vi "Drive output parameters.vi"   [LabVIEW 2016]
uses:
  Robot Global Data.vi
types:
  T1 = enum16{"FL Drive Wheel", "FR Drive Wheel", "RL Drive Wheel", "RR Drive Wheel", "FL Steer Wheel", "FR Steer Wheel", "RL Steer Wheel", "RR Steer Wheel"}
  T2 = typedef "WPI_MotorControlDeviceRef.ctl" = cluster{"DeviceStatus":errorcluster, "Type":T3, "PWM":cluster{"PWM Channel":T4, "DeadBand":T5}, "CAN":cluster{"Device Number":u8, "SetOutput VI Ref":variant, "GetOutput VI Ref":variant, "Enable VI Ref":variant, "Disable VI Ref":variant, "Data":variant}, "Invert":bool}
  T3 = typedef "WPI_MotorControlType.ctl" = enum16{"PWM", "CAN"}
  T4 = typedef "FPGA_DIOPWMChannel.ctl" = enum8{"PWM 0", "PWM 1", "PWM 2", "PWM 3", "PWM 4", "PWM 5", "PWM 6", "PWM 7", "PWM 8", "PWM 9", "PWM MXP 0", "PWM MXP 1", "PWM MXP 2", "PWM MXP 3", "PWM MXP 4", "PWM MXP 5", "PWM MXP 6", "PWM MXP 7", "PWM MXP 8", "PWM MXP 9", "Invalid"}
  T5 = typedef "WPI_PWMDeadband.ctl" = cluster{"Name":string, "maxPositivePwm":i32, "minPositivePwm":i32, "centerPwm":i32, "maxNegativePwm":i32, "minNegativePwm":i32, "angularRange":u16}
  T6 = typedef "WPI_CANTalonSRX_GlobalStatus.ctl" = cluster{"Applied Throttle":dbl, "Module Enabled":bool, "CAN Error":errorcluster, "Closed Loop Error":dbl, "Forward Limit Switch Closed":bool, "Reverse Limit Switch Closed":bool, "Sensor Position":dbl, "Sensor Velocity":dbl, "Current":dbl, "Sticky Fault - Over Temp":bool, "Sticky Fault - Under Voltage":bool, "Sticky Fault - Forward Limit":bool, "Sticky Fault - Reverse Limit":bool, "Sticky Fault - Forward Soft Limit":bool, "Sticky Fault - Reverse Soft Limit":bool, "Brake is Enabled":bool, "Encoder Position":dbl, "Encoder Velocity":dbl, "Encoder Index Count":dbl, "Encoder A Pin State":bool, "Encoder B Pin State":bool, "Encoder Index Pin State":bool, "Analog In":dbl, "Analog In Velocity":dbl, "Temperature (C)":dbl, "Battery Voltage":dbl, "Control 5 Is Supported":bool, "Current Profile Slot Select":dbl, "Pos Div 8":bool, "Vel Div 4":bool, "Pulse Width Position":i32, "Pulse Width Velocity":i32, "Pulse Width Rise To Rise (us)":i32, "Pulse Width Rise To Fall (us)":i32, "Mot Prof Active Is Under Run":bool, "Mot Prof Active Has Under Run":bool, "Mot Prof Active Is Last":bool, "Mot Prof Active Velocity Only":bool, "Mot Prof Active Is Valid":bool, "Mot Prof Buffer Is Full":bool, "Mot Prof Active Profile Slot Select":i32, "Mot Prof NextID":i32, "Mot Prof Count":i32, "Mot Prof Active Velocity":dbl, "Mot Prof Active Position":dbl, "Mot Prof Output Enable":i32}
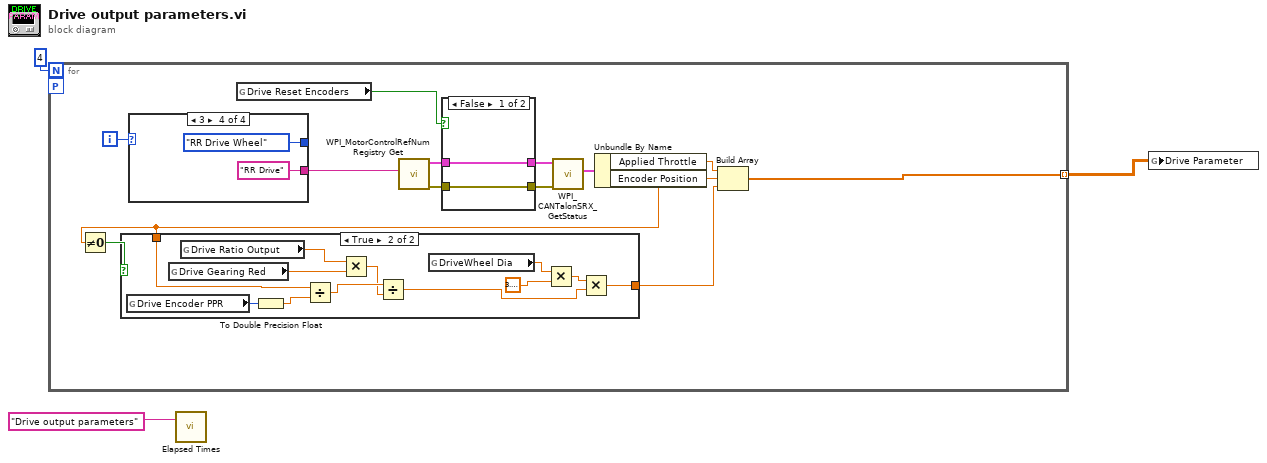
[diagram p0: block diagram]
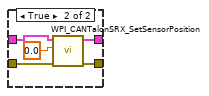
[diagram p3: hidden frame]
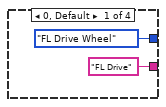
[diagram p4: hidden frame]
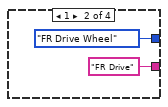
[diagram p5: hidden frame]
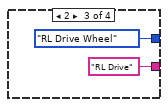
[diagram p6: hidden frame]
diagram:
  n1 = for {
    N: 4 -> [_]
    tunnel: [w12] -> w2 mode=indexing
    workers-P: _ -> [_]
    i -> [w16]
    n2 = case shown="3" w16 {
      tunnel: [T1."FL Drive Wheel" ("Swerve Drive Param") T1."FR Drive Wheel" ("Swerve Drive Param") T1."RL Drive Wheel" ("Swerve Drive Param") T1."RR Drive Wheel" ("Swerve Drive Param")] -> _
      tunnel: ["FL Drive" ("refnum name") "FR Drive" ("refnum name") "RL Drive" ("refnum name") "RR Drive" ("refnum name")] -> w14
      frame 0, Default {
      }
      frame 1 {
      }
      frame 2 {
      }
      frame 3 {
      }
    }
    n3 = global read "Robot Global Data.vi" "Drive Reset Encoders"() -> (w7:bool)
    n4 = call <vilib>:"WPI_MotorControlRefNum Registry Get.vi"("refnum name"=w14) -> ("error out"=w11:errorcluster, "MotorControlDevRef"=w10:T2)  [unwired: 9 in]
    n5 = case shown="False" w7 {
      tunnel: w11 -> [w30 w36]
      tunnel: w10 -> [w31 w35]
      tunnel: [w31 w34] -> w9
      tunnel: [w30 w33] -> w8
      frame False {
      }
      frame True {
        n6 = call <vilib>:"WPI_CANTalonSRX_SetSensorPosition.vi"("error in (no error)"=w36, "New Sensor Position"=0.0, "CAN Talon SRX Ref"=w35) -> ("error out"=w33:errorcluster, "CAN Talon SRX Ref"=w34:T2)  [unwired: 7 in]
      }
    }
    n7 = call <vilib>:"WPI_CANTalonSRX_GetStatus.vi"("error in (no error)"=w8, "CAN Talon SRX Ref"=w9) -> ("Talon SRX Status"=w15:T6)  [unwired: 7 in, 2 out]
    n8 = Unbundle By Name(w15) -> ("Applied Throttle"=w13:dbl, "Encoder Position"=w4:dbl)
    n9 = Not Equal To 0?(x=w4) -> (x != 0?=w6:bool)
    n10 = case shown="True" w6 {
      tunnel: w4 -> [w17 w28]
      tunnel: [w17 w22] -> w5
      frame False {
      }
      frame True {
        n11 = global read "Robot Global Data.vi" "Drive Encoder PPR"() -> (w29:u32)
        n12 = global read "Robot Global Data.vi" "Drive Gearing Red"() -> (w20:dbl)
        n13 = global read "Robot Global Data.vi" "Drive Ratio Output"() -> (w21:dbl)
        n14 = To Double Precision Float(number=w29) -> (double precision float=w27:dbl)
        n15 = Divide(x=w28, y=w27) -> (x/y=w19:dbl)
        n16 = Multiply(x=w21, y=w20) -> (x*y=w18:dbl)
        n17 = Divide(x=w19, y=w18) -> (x/y=w23:dbl)
        n18 = global read "Robot Global Data.vi" "DriveWheel Dia"() -> (w26:dbl)
        n19 = Multiply(x=w26, y=3.141592653589793) -> (x*y=w24:dbl)
        n20 = Multiply(x=w24, y=w23) -> (x*y=w22:dbl)
      }
    }
    n21 = Build Array(w13, w4, w5) -> (w12:dbl[])
  }
  n22 = call "Elapsed Times.vi"("Call Name"="Drive output parameters") -> ()  [unwired: 2 in, 1 out]
  n23 = global write "Robot Global Data.vi" "Drive Parameter"(w2) -> ()
